vi "ModifyPressures.vi"(6 "Ctr Pressure In":dbl=292.8560256927093, 8 "Pressure For Mix 2":dbl[](array[numeric]), 9 "Pressure For Mix 1":dbl[](array[numeric]), 11 "Mix Cluster":T1={"Ratio"=[0.6, 0.5], "Mix 2"=[12, 12], "Mix 1"=[0, 1]} {"Mix 1" items=["A1"=0, "A2"=1, "A3"=2, "A4"=3, "A5"=12]; "Mix 2" items=["B5"=8, "B6"=9, "B7"=10, "B8"=11, "A5"=12]}) -> (0 "Modified Pressure for Mix 2":dbl[](array[numeric]), 1 "Modified Pressure for Mix 1":dbl[](array[numeric]), 4 "Control Pressure Out":dbl)   [LabVIEW 2016]
uses:
  Labjack/ValveGlobals.vi
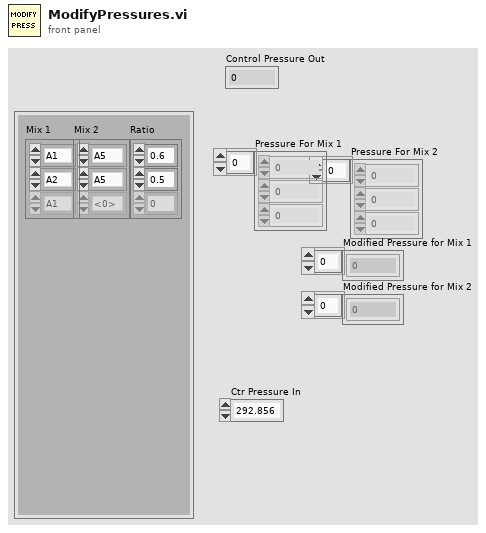
[diagram p1: front panel]
types:
  T1 = cluster{"Ratio":dbl[], "Mix 2":u16[], "Mix 1":u16[]}
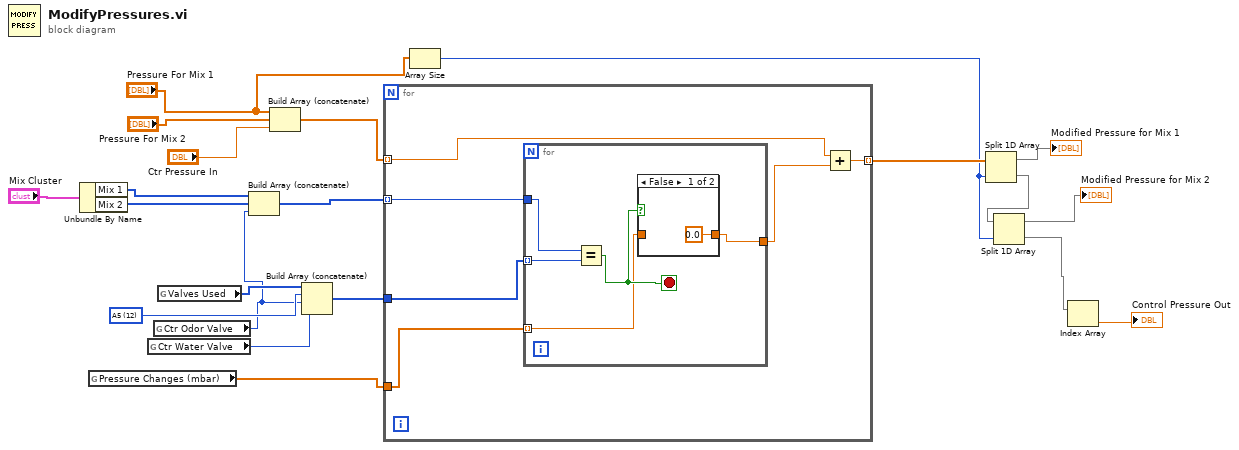
[diagram p0: block diagram]
diagram:
  w19 = u16 12 items=["A1", "A2", "A3", "A4", "B1", "B2", "B3", "B4", "B5", "B6", "B7", "B8", "A5", "A6", "A7", "A8"] ("Ctr Odor Valve")
  n1 = Unbundle By Name("Mix Cluster") -> ("Mix 1"=w17:u16[], "Mix 2"=w16:u16[])
  n2 = global read "ValveGlobals.vi" "Pressure Changes (mbar)"() -> (w12:dbl[])
  n3 = global read "ValveGlobals.vi" "Ctr Water Valve"() -> (w3:u16)
  n4 = global read "ValveGlobals.vi" "Ctr Odor Valve"() -> (w7:u16)
  n5 = global read "ValveGlobals.vi" "Valves Used"() -> (w20:u16[])
  n6 = Build Array (concatenate)(w17, w16, w7) -> (w15:u16[])
  n7 = Build Array (concatenate)("Pressure For Mix 1", "Pressure For Mix 2", "Ctr Pressure In") -> (w14:dbl[])
  n8 = Build Array (concatenate)(w20, w19, w7, w3) -> (w13:u16[])
  n9 = for {
    tunnel: w15 -> [w26] mode=indexing
    tunnel: w14 -> [w23] mode=indexing
    tunnel: w13 -> [w27]
    tunnel: w12 -> [w25]
    tunnel: [w22] -> w11 mode=indexing
    n10 = for {
      tunnel: w27 -> [w31] mode=indexing
      tunnel: w26 -> [w32]
      tunnel: w25 -> [w29] mode=indexing
      tunnel: [w28] -> w24
      stop <- w30 stop-if-true
      n11 = Equal?(x=w32, y=w31) -> (x = y?=w30:bool)
      n12 = case shown="False" w30 {
        tunnel: w29 -> [_ w34]
        tunnel: [0.0 w34] -> w28
        frame False {
        }
        frame True {
        }
      }
    }
    n13 = Add(x=w23, y=w24) -> (x+y=w22:dbl)
  }
  n14 = Array Size(array="Pressure For Mix 1") -> (size(s)=w5:i32)
  n15 = Split 1D Array(array=w11, index=w5) -> (first subarray=→"Modified Pressure for Mix 1":dbl[], second subarray=w6:dbl[])
  n16 = Split 1D Array(array=w6, index=w5) -> (first subarray=→"Modified Pressure for Mix 2":dbl[], second subarray=w2:dbl[])
  n17 = Index Array(array=w2) -> (element=→"Control Pressure Out":dbl)  [unwired: 1 in]
